vi "Set-framegrabber-status.vi"(8 "error in":errorcluster, 9 "Reset errors?":bool, 10 "Grabber status in":T1=enum."Active", 11 "Data ref. in":refnum<data-value>) -> (0 "error IO":errorcluster, 2 "Grabber status":T1, 3 "Data ref.":refnum<data-value>)   [LabVIEW 2013, in "CameraVision.lvlib" / "CV-Main.lvclass"]
doc: "This function loads the default values for the hidden program parameters from an .xml file and writes these values to the parameter groups.\nThe file path for the hidden parameters is '<Application directory>\\Program data\\parameters-hidden.xml'.\nThe hidden parameters can not be changed through the CameraVision program, but can be changed using the 'CV-Set-hidden-parameters.vi' utility."
uses:
  CV-Main.lvclass
  UI/Module-states.ctl
  CV-Main.lvclass/CV-Main.ctl
  Configuration/CV-Configuration.lvclass/CV-Configuration.ctl
  Read Config params.vi
  Configuration/Read Grabber status.vi
  Configuration/Write Grabber status.vi
  Configuration/CV-Configuration.lvclass
  UI/CV-UI.lvclass
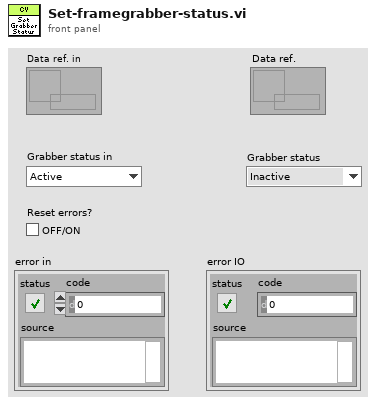
[diagram p1: front panel]
types:
  T1 = typedef "CameraVision.lvlib/CV-UI.lvclass/Module-states.ctl" = enum16{"Inactive", "Active", "Data-loss", "Error", "Simulation", "Synchronizing", "Initialized", "Released"}
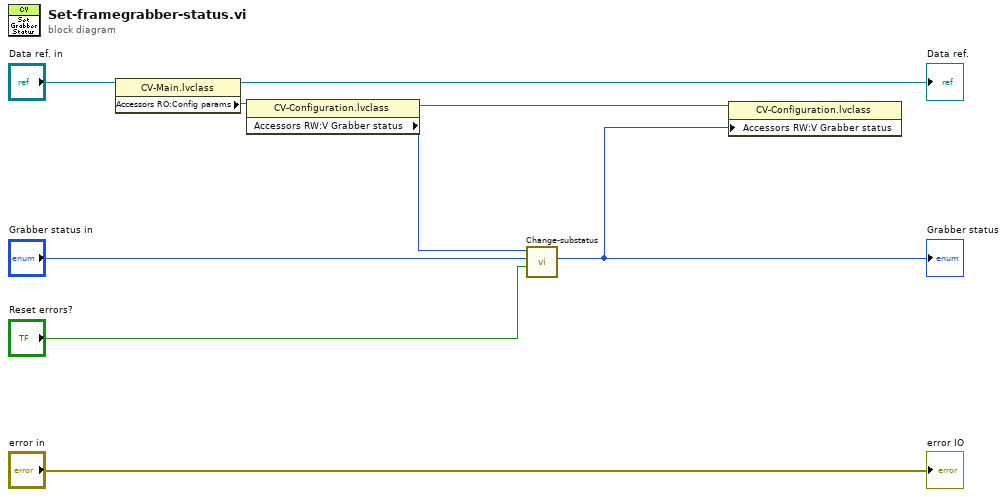
[diagram p0: block diagram]
diagram:
  n1 = property class="CV-Main.lvclass"(reference="Data ref. in") -> (reference out=→"Data ref.":refnum<data-value>, "Accessors RO:Config params"=w3:refnum<data-value>)  [unwired: 1 in, 1 out]
  n2 = property class="CV-Configuration.lvclass"(reference=w3) -> (reference out=w1:refnum<data-value>, "Accessors RW:V Grabber status"=w2:T1)  [unwired: 1 in, 1 out]
  n3 = call "Change-substatus.vi"("Reset errors?"="Reset errors?", "New status in"="Grabber status in", "Previous status"=w2) -> ("New status"=w4:T1)  [unwired: 8 in]
  "Grabber status" <- w4
  n4 = property class="CV-Configuration.lvclass"(reference=w1, "Accessors RW:V Grabber status"=w4) -> ()  [unwired: 1 in, 2 out]
  "error IO" <- "error in"
